vi "FTW-ProjectManager-GetProjectPath.vi"(0 "Project Manager":refnum<class "FTW-ProjectManager.lvclass">, 11 "error in":errorcluster) -> (4 "Project Manager out":refnum<class "FTW-ProjectManager.lvclass">, 6 "Project Filepath":path, 8 "Project Directory":path, 15 "error out":errorcluster)   [LabVIEW 2012, in "FTW-ProjectManager.lvclass"]
uses:
  FTW-ProjectManager.lvclass
  FTW-ProjectManager.lvclass/FTW-ProjectManager.ctl
panel:
  # "Inputs"
  # "Outputs"
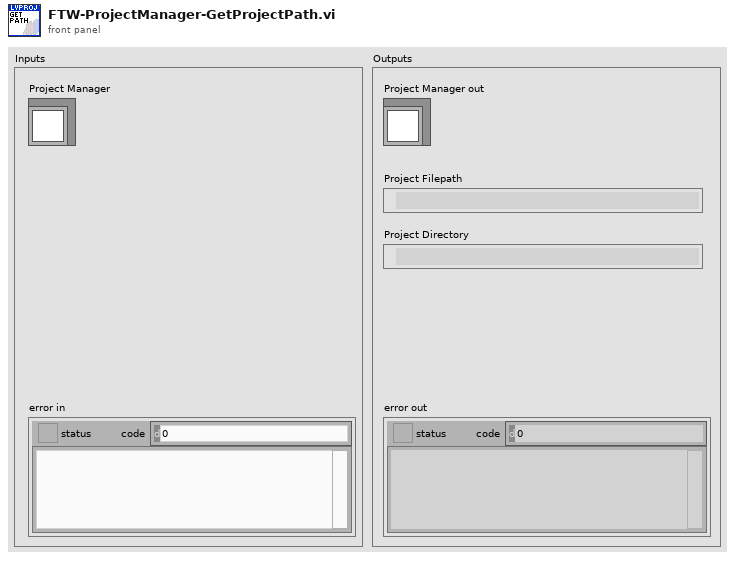
[diagram p1: front panel]
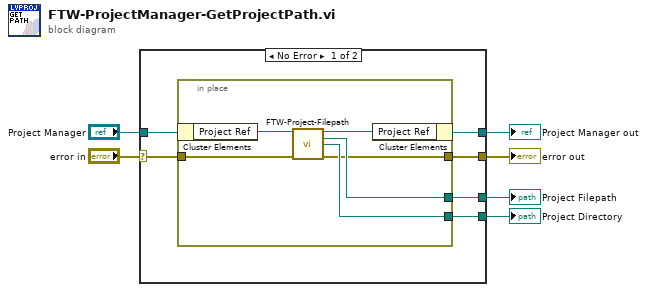
[diagram p0: block diagram]
diagram:
  n1 = case shown="No Error" "error in" {
    selector: "error in" -> [w10 w20]
    tunnel: [w9 w20] -> w6
    tunnel: [w7 w19] -> w4
    tunnel: "Project Manager" -> [w8 w19]
    tunnel: [w12 _] -> w2
    tunnel: [w11 _] -> w1
    frame No Error {
      n2 = in-place {
        in-place-border: [w18] -> w12
        in-place-border: [w17] -> w11
        in-place-border: w10 -> [w16]
        in-place-border: [w15] -> w9
        n3 = in-place-cluster #1(w8) -> ("Project Ref"=w14:refnum<vi>)
        n4 = call "FTW-Project-Filepath.vi"("Project Ref"=w14, "error in"=w16) -> ("Project Ref out"=w13:refnum<vi>, "Project Filepath"=w18:path, "Project Directory"=w17:path, "error out"=w15:errorcluster)  [unwired: 10 in]
        n5 = in-place-cluster #1("Project Ref"=w13) -> (w7:refnum<class "FTW-ProjectManager.lvclass">)
      }
    }
    frame Error {
    }
  }
  "error out" <- w6
  "Project Manager out" <- w4
  "Project Filepath" <- w2
  "Project Directory" <- w1
